vi "Stop Core.vi"(10 "final error code":i32, 11 "Water Level in":refnum<class "Water Level.lvclass">) -> (3 "Water Level out":refnum<class "Water Level.lvclass">)   [LabVIEW 2012, in "Water Level.lvclass"]
doc: "(<B>Filename</B>: Actor Framework.lvlib:Actor.lvclass:Stop Core.vi)\n\nDefines what the actor does before it stops. Use the <B>final error code</B> input to determine whether the actor shut down in response to an error.\n\nBy default, this method does nothing. A descendant class may override it to define behavior, such as shutting down any processes the actor initiated in its override of the Actor Core method."
uses:
  Water Level.lvclass
  Level Controller/Level Controller/Level Controller.lvclass
  Simulation/Simulation Data_Global.vi
  Simulation/Simulation.lvlib
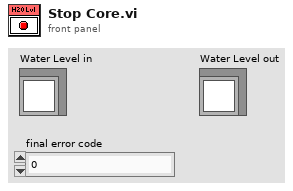
[diagram p1: front panel]
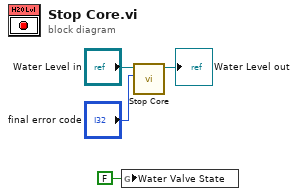
[diagram p0: block diagram]
diagram:
  n1 = global write "Simulation Data_Global.vi" "Water Valve State"(FALSE ("Water Valve State")) -> ()
  n2 = call-parent "Stop Core.vi"("final error code"="final error code", "Actor in"="Water Level in") -> ("Actor out"=→"Water Level out":refnum<class "Water Level.lvclass">)  [unwired: 9 in]
